vi "Rotate_Images.vi"(8 "Rotated Dst 2":T1, 9 "Image Src 2":T1, 10 "Rotated Dst 1":T1, 11 "Image Src 1":T1) -> (1 "Rotated Image 2":T1, 2 "Rotated Image 1":T1)   [LabVIEW 2011]
uses:
  <vilib>/vision/Image Controls.llb/IMAQ Image.ctl
  <vilib>/vision/NI_Vision_Development_Module.lvlib
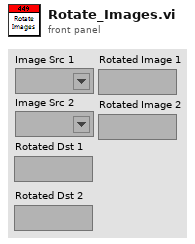
[diagram p1: front panel]
types:
  T1 = typedef "IMAQ Image.ctl" = refnum<image>
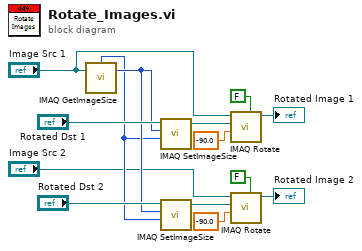
[diagram p0: block diagram]
diagram:
  n1 = call "IMAQ GetImageSize"("Image"="Image Src 1") -> ("Y Resolution"=w12:i32, "X Resolution"=w11:i32)  [unwired: 3 in, 1 out]
  n2 = call "IMAQ SetImageSize"("Y Resolution"=w11, "X Resolution"=w12, "Image"="Rotated Dst 1") -> ("Image Out"=w9:T1)  [unwired: 2 in, 1 out]
  n3 = call "IMAQ SetImageSize"("Y Resolution"=w11, "X Resolution"=w12, "Image"="Rotated Dst 2") -> ("Image Out"=w4:T1)  [unwired: 2 in, 1 out]
  n4 = call "IMAQ Rotate"("Maintain Size"=FALSE, "Angle (degrees)"=sgl -90.0, "Image Dst"=w9, "Image Src"="Image Src 1") -> ("Image Dst Out"=→"Rotated Image 1":T1)  [unwired: 6 in, 1 out]
  n5 = call "IMAQ Rotate"("Maintain Size"=FALSE, "Angle (degrees)"=sgl -90.0, "Image Dst"=w4, "Image Src"="Image Src 2") -> ("Image Dst Out"=→"Rotated Image 2":T1)  [unwired: 6 in, 1 out]
